vi "JSONHandler.vi"(0 "params":variant, 1 "JSON-response":string, 2 "rpc":string="2.0", 3 "method":string, 5 "ID":string="1", 8 "Set":bool) -> (14 "result":variant, 15 "JSON-request":string, 16 "rpc":string, 17 "method":string, 19 "ID":string)   [LabVIEW 2016]
uses:
  <vilib>/Utility/Data Type/NI_Data Type.lvlib
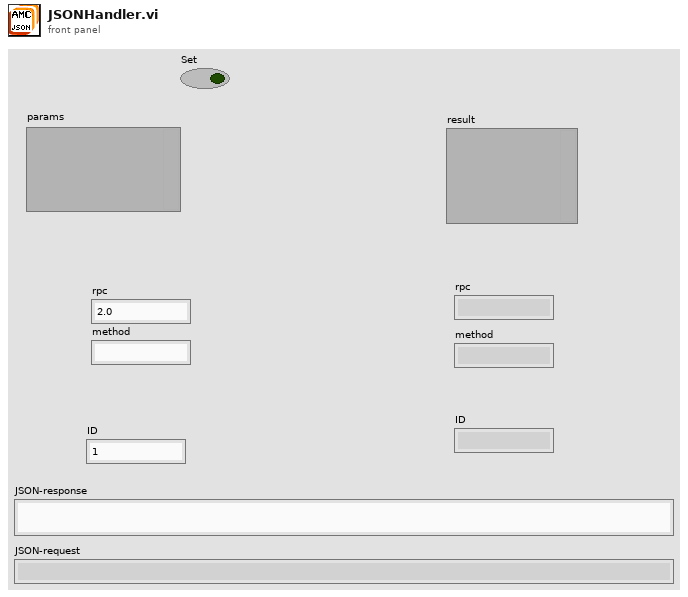
[diagram p1: front panel]
types:
  T1 = cluster{"jsonrpc":string, "method":string, "params":i32[], "id":string}
  T2 = cluster{"jsonrpc":string, "method":string, "params":string[], "id":string}
  T3 = cluster{"jsonrpc":string, "method":string, "params":bool[], "id":string}
  T4 = typedef "NI_Data Type.lvlib/Data Type.ctl" = enum8{"Invalid Type", "Void", "I8", "I16", "I32", "I64", "U8", "U16", "U32", "U64", "Single Float", "Double Float", "Extended Float", "Single Complex", "Double Complex", "Extended Complex", "Enum U8", "Enum U16", "Enum U32", "Enum U64", "Single Float With Unit", "Double Float With Unit", "Extended Float With Unit", "Single Complex with Unit", "Double Complex with Unit", "Extended Complex with Unit", "Boolean", "String", "Path", "Picture", "Tag", "Array", "Cluster", "Variant", "LV Variant", "Waveform", "Timestamp", "Digital Waveform", "Digital Data", "ExpressData", "Refnum", "External Data", "VI", "Poly VI", "LabVIEW Class Instance", "Fixed Point"}
  T5 = cluster{"Cluster Elements[0]":variant, "Cluster Elements[1]":variant}
  T6 = cluster{"Cluster Elements[0]":variant, "Cluster Elements[1]":variant, "Cluster Elements[2]":variant}
  T7 = cluster{"Cluster Elements[0]":variant, "Cluster Elements[1]":variant, "Cluster Elements[2]":variant, "Cluster Elements[3]":variant}
  T8 = cluster{"Cluster Elements[0]":variant, "Cluster Elements[1]":variant, "Cluster Elements[2]":variant, "Cluster Elements[3]":variant, "Cluster Elements[4]":variant}
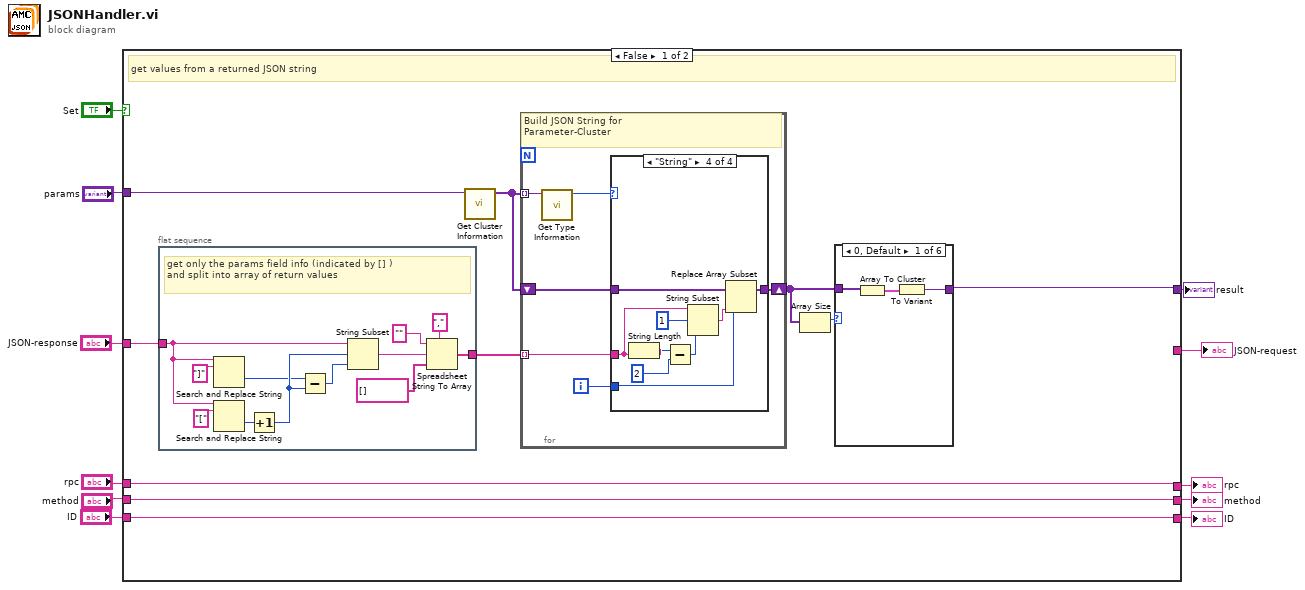
[diagram p0: block diagram]
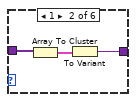
[diagram p2: hidden frame]
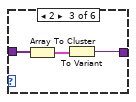
[diagram p3: hidden frame]
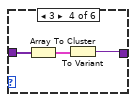
[diagram p4: hidden frame]
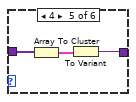
[diagram p5: hidden frame]
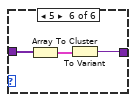
[diagram p6: hidden frame]
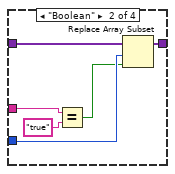
[diagram p8: hidden frame]
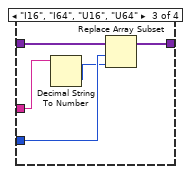
[diagram p9: hidden frame]
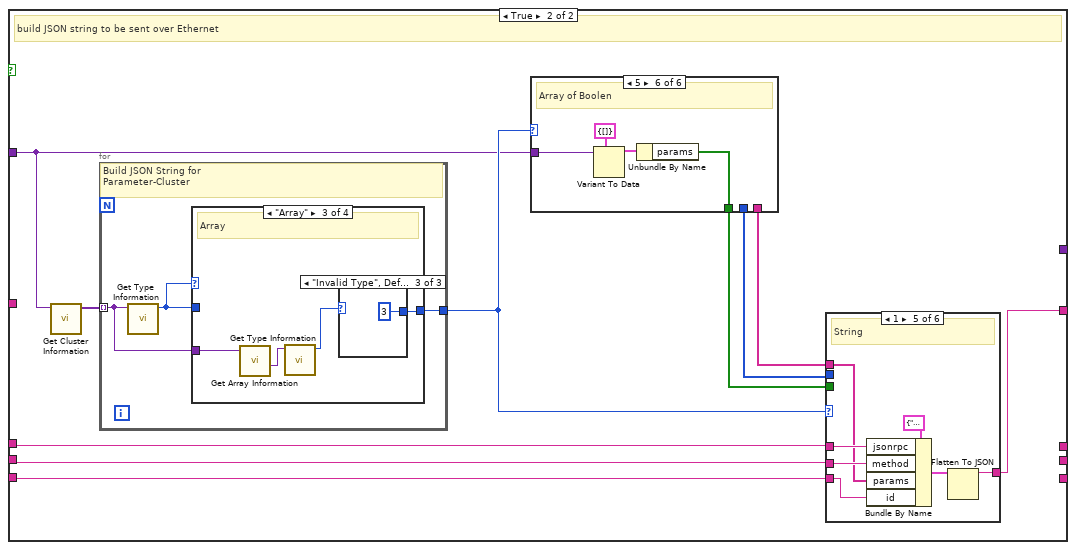
[diagram p10: hidden frame]
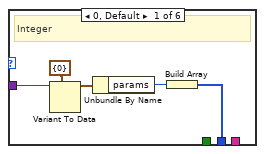
[diagram p11: hidden frame]
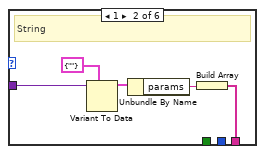
[diagram p12: hidden frame]
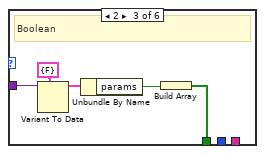
[diagram p13: hidden frame]
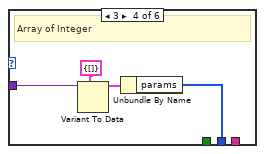
[diagram p14: hidden frame]
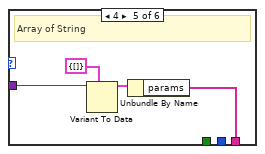
[diagram p15: hidden frame]
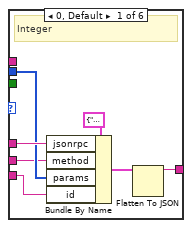
[diagram p16: hidden frame]
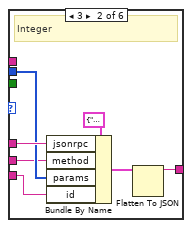
[diagram p17: hidden frame]
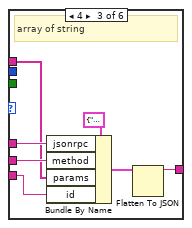
[diagram p18: hidden frame]
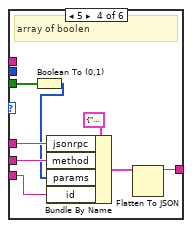
[diagram p19: hidden frame]
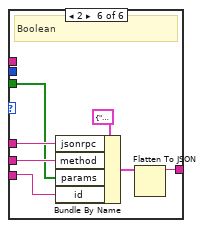
[diagram p20: hidden frame]
diagram:
  n1 = case shown="False" "Set" {
    tunnel: "JSON-response" -> [w21 _]
    tunnel: "params" -> [w12 w83]
    tunnel: [w17 _] -> w2
    tunnel: [w16 _] -> w8
    tunnel: "method" -> [w16 w81]
    tunnel: "rpc" -> [w15 w82]
    tunnel: [w15 _] -> w6
    tunnel: "ID" -> [w14 w80]
    tunnel: [w14 _] -> w4
    tunnel: [_ w79] -> w3
    frame False {
      # "get values from a returned JSON string"
      n2 = flat-sequence {
        tunnel: [w41] -> w13
        tunnel: w21 -> [w40]
        frame #0 {
          # "get only the params field info (indicated by [] )\nand split into array of return values"
          n3 = Search and Replace String(input string=w40, search string="]") -> (offset past replacement=w44:i32)  [unwired: 6 in, 3 out]
          n4 = Search and Replace String(input string=w40, search string="[") -> (offset past replacement=w45:i32)  [unwired: 6 in, 3 out]
          n5 = Increment(x=w45) -> (x+1=w46:i32)
          n6 = Subtract(x=w44, y=w46) -> (x-y=w47:i32)
          n7 = String Subset(string=w40, offset (0)=w46, length (rest)=w47) -> (substring=w48:string)
          n8 = Spreadsheet String To Array(delimiter (Tab)="," ("spreadsheet string"), format string="", spreadsheet string=w48, array type (2D Dbl)=string[] []) -> (array=w41:string[])
        }
      }
      n9 = call <vilib>:"Get Cluster Information.vi"("Variant"=w12) -> ("Cluster Elements"=w20:variant[])  [unwired: 9 in, 1 out]
      n10 = for {
        tunnel: w13 -> [w52] mode=indexing
        tunnel: w20 -> [w57] mode=indexing
        shift-right: [w54] -> w18
        shift-left: w20 -> [w55]
        i -> [w53]
        # "Build JSON String for \nParameter-Cluster"
        n11 = call <vilib>:"Get Type Information.vi"("Variant"=w57) -> ("Type"=w56:T4)  [unwired: 6 in, 4 out]
        n12 = case shown="\"String\"" w56 {
          tunnel: w55 -> [w58 w63 w69 w78]
          tunnel: [w58 w62 w68 w77] -> w54
          tunnel: w53 -> [_ w60 w67 w76]
          tunnel: w52 -> [_ w61 w66 w73]
          frame "Invalid Type", Default {
          }
          frame "Boolean" {
            n13 = Equal?(x=w61, y="true") -> (x = y?=w59:bool)
            n14 = Replace Array Subset(array=w63, new element=w59, index=w60) -> (w62:variant[])
          }
          frame "I16", "I64", "U16", "U64" {
            n15 = Decimal String To Number(string=w66) -> (number=w65:i32)  [unwired: 2 in, 1 out]
            n16 = Replace Array Subset(array=w69, new element=w65, index=w67) -> (w68:variant[])
          }
          frame "String" {
            n17 = String Length(string=w73) -> (length=w71:i32)
            n18 = Subtract(x=w71, y=2 ("offset (0)")) -> (x-y=w70:i32)
            n19 = String Subset(string=w73, offset (0)=1, length (rest)=w70) -> (substring=w74:string)
            n20 = Replace Array Subset(array=w78, new element=w74, index=w76) -> (w77:variant[])
          }
        }
      }
      n21 = Array Size(array=w18) -> (size(s)=w19:i32)
      n22 = case shown="0, Default" w19 {
        tunnel: w18 -> [w23 w26 w29 w32 w35 w38]
        tunnel: [w22 w25 w28 w31 w34 w37] -> w17
        frame 0, Default {
          n23 = Array To Cluster(array=w23) -> (cluster=w24:cluster{"Cluster Elements[0]":variant})
          n24 = To Variant(anything=w24) -> (Variant=w22:variant)
        }
        frame 1 {
          n25 = Array To Cluster(array=w26) -> (cluster=w27:cluster{"Cluster Elements[0]":variant})
          n26 = To Variant(anything=w27) -> (Variant=w25:variant)
        }
        frame 2 {
          n27 = Array To Cluster(array=w29) -> (cluster=w30:T5)
          n28 = To Variant(anything=w30) -> (Variant=w28:variant)
        }
        frame 3 {
          n29 = Array To Cluster(array=w32) -> (cluster=w33:T6)
          n30 = To Variant(anything=w33) -> (Variant=w31:variant)
        }
        frame 4 {
          n31 = Array To Cluster(array=w35) -> (cluster=w36:T7)
          n32 = To Variant(anything=w36) -> (Variant=w34:variant)
        }
        frame 5 {
          n33 = Array To Cluster(array=w38) -> (cluster=w39:T8)
          n34 = To Variant(anything=w39) -> (Variant=w37:variant)
        }
      }
    }
    frame True {
      # "build JSON string to be sent over Ethernet"
      n35 = call <vilib>:"Get Cluster Information.vi"("Variant"=w83) -> ("Cluster Elements"=w84:variant[])  [unwired: 9 in, 1 out]
      n36 = for {
        tunnel: w84 -> [w159] mode=indexing
        tunnel: [w161] -> w85
        # "Build JSON String for \nParameter-Cluster"
        n37 = call <vilib>:"Get Type Information.vi"("Variant"=w159) -> ("Type"=w160:T4)  [unwired: 6 in, 4 out]
        n38 = case shown="\"Array\"" w160 {
          tunnel: w160 -> [_ _ _ _]
          tunnel: [1 2 w167 0] -> w161
          tunnel: w159 -> [_ _ w165 _]
          frame "String" {
            # "String"
          }
          frame "Boolean" {
            # "Boolean"
          }
          frame "Array" {
            # "Array"
            n39 = call <vilib>:"Get Array Information.vi"("Variant"=w165) -> ("Array Element Data Type"=w164:variant)  [unwired: 7 in, 3 out]
            n40 = call <vilib>:"Get Type Information.vi"("Variant"=w164) -> ("Type"=w166:T4)  [unwired: 6 in, 4 out]
            n41 = case shown="\"Invalid Type\", Default" w166 {
              tunnel: [4 5 3] -> w167
              frame "String" {
              }
              frame "Boolean" {
              }
              frame "Invalid Type", Default {
              }
            }
          }
          frame "Invalid Type", Default {
            # "Integer"
          }
        }
      }
      n42 = case shown="5" w85 {
        tunnel: w83 -> [w91 w97 w101 w105 w109 w113]
        tunnel: [w89 _ _ w104 _ _] -> w88
        tunnel: [_ w94 _ _ w108 _] -> w87
        tunnel: [_ _ w99 _ _ w112] -> w86
        frame 0, Default {
          # "Integer"
          n43 = Variant To Data(type=cluster{"params":i32} {"params"=0} ("input cluster"), Variant=w91) -> (data=w92:cluster{"params":i32})  [unwired: 1 in, 1 out]
          n44 = Unbundle By Name(w92) -> ("params"=w90:i32)
          n45 = Build Array(w90) -> (w89:i32[])
        }
        frame 1 {
          # "String"
          n46 = Variant To Data(type=cluster{"params":string} {"params"=""} ("input cluster"), Variant=w97) -> (data=w96:cluster{"params":string})  [unwired: 1 in, 1 out]
          n47 = Unbundle By Name(w96) -> ("params"=w95:string)
          n48 = Build Array(w95) -> (w94:string[])
        }
        frame 2 {
          # "Boolean"
          n49 = Variant To Data(type=cluster{"params":bool} {"params"=FALSE} ("input cluster"), Variant=w101) -> (data=w102:cluster{"params":bool})  [unwired: 1 in, 1 out]
          n50 = Unbundle By Name(w102) -> ("params"=w100:bool)
          n51 = Build Array(w100) -> (w99:bool[])
        }
        frame 3 {
          # "Array of Integer"
          n52 = Variant To Data(type=cluster{"params":i32[]} {"params"=[]} ("input cluster"), Variant=w105) -> (data=w106:cluster{"params":i32[]})  [unwired: 1 in, 1 out]
          n53 = Unbundle By Name(w106) -> ("params"=w104:i32[])
        }
        frame 4 {
          # "Array of String"
          n54 = Variant To Data(type=cluster{"params":string[]} {"params"=[]} ("input cluster"), Variant=w109) -> (data=w110:cluster{"params":string[]})  [unwired: 1 in, 1 out]
          n55 = Unbundle By Name(w110) -> ("params"=w108:string[])
        }
        frame 5 {
          # "Array of Boolen"
          n56 = Variant To Data(type=cluster{"params":bool[]} {"params"=[]} ("input cluster"), Variant=w113) -> (data=w114:cluster{"params":bool[]})  [unwired: 1 in, 1 out]
          n57 = Unbundle By Name(w114) -> ("params"=w112:bool[])
        }
      }
      n58 = case shown="1" w85 {
        tunnel: w82 -> [w122 w129 w136 w144 w150 w156]
        tunnel: w81 -> [w117 w124 w132 w140 w149 w155]
        tunnel: [w119 w126 w133 w141 w147 w153] -> w79
        tunnel: w88 -> [w118 w125 _ _ _ _]
        tunnel: w87 -> [_ _ w130 _ w146 _]
        tunnel: w86 -> [_ _ _ w138 _ w154]
        tunnel: w80 -> [w116 w123 w131 w139 w145 w152]
        frame 0, Default {
          # "Integer"
          n59 = Bundle By Name(cluster=T1 {"jsonrpc"="", "method"="", "params"=[], "id"=""} ("anything"), "jsonrpc"=w122, "method"=w117, "params"=w118, "id"=w116) -> (w120:T1)
          n60 = Flatten To JSON(anything=w120) -> (JSON string=w119:string)  [unwired: 2 in, 1 out]
        }
        frame 3 {
          # "Integer"
          n61 = Bundle By Name(cluster=T1 {"jsonrpc"="", "method"="", "params"=[], "id"=""} ("anything"), "jsonrpc"=w129, "method"=w124, "params"=w125, "id"=w123) -> (w127:T1)
          n62 = Flatten To JSON(anything=w127) -> (JSON string=w126:string)  [unwired: 2 in, 1 out]
        }
        frame 4 {
          # "array of string"
          n63 = Bundle By Name(cluster=T2 {"jsonrpc"="", "method"="", "params"=[], "id"=""} ("anything"), "jsonrpc"=w136, "method"=w132, "params"=w130, "id"=w131) -> (w134:T2)
          n64 = Flatten To JSON(anything=w134) -> (JSON string=w133:string)  [unwired: 2 in, 1 out]
        }
        frame 5 {
          # "array of boolen"
          n65 = Boolean To (0,1)(Boolean=w138) -> (0, 1=w137:i16[])
          n66 = Bundle By Name(cluster=T1 {"jsonrpc"="", "method"="", "params"=[], "id"=""} ("anything"), "jsonrpc"=w144, "method"=w140, "params"=w137, "id"=w139) -> (w142:T1)
          n67 = Flatten To JSON(anything=w142) -> (JSON string=w141:string)  [unwired: 2 in, 1 out]
        }
        frame 1 {
          # "String"
          n68 = Bundle By Name(cluster=T2 {"jsonrpc"="", "method"="", "params"=[], "id"=""} ("anything"), "jsonrpc"=w150, "method"=w149, "params"=w146, "id"=w145) -> (w148:T2)
          n69 = Flatten To JSON(anything=w148) -> (JSON string=w147:string)  [unwired: 2 in, 1 out]
        }
        frame 2 {
          # "Boolean"
          n70 = Bundle By Name(cluster=T3 {"jsonrpc"="", "method"="", "params"=[], "id"=""} ("anything"), "jsonrpc"=w156, "method"=w155, "params"=w154, "id"=w152) -> (w158:T3)
          n71 = Flatten To JSON(anything=w158) -> (JSON string=w153:string)  [unwired: 2 in, 1 out]
        }
      }
    }
  }
  "result" <- w2
  "method" <- w8
  "rpc" <- w6
  "ID" <- w4
  "JSON-request" <- w3
